vi "LVProjectShortcut_CreateNewWizard_Invoke.vi"(10 "Cluster":T1, 11 "Wizard":T2) -> (3 "Canceled":bool)   [LabVIEW 2017]
uses:
  <resource>/Framework/Providers/API/ItemRef.ctl
  <resource>/Framework/Providers/API/mxLvNIIM.ctl
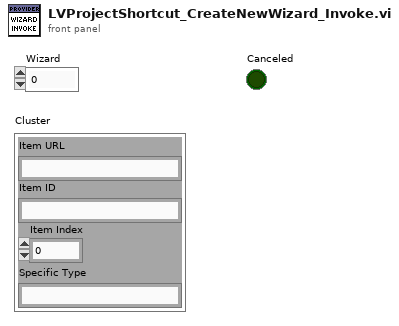
[diagram p1: front panel]
types:
  T1 = typedef "mxLvNIIM.ctl" = cluster{"Item URL":string, "Item ID":string, "Item Index":i32, "Specific Type":string}
  T2 = typedef "ItemRef.ctl" = u64
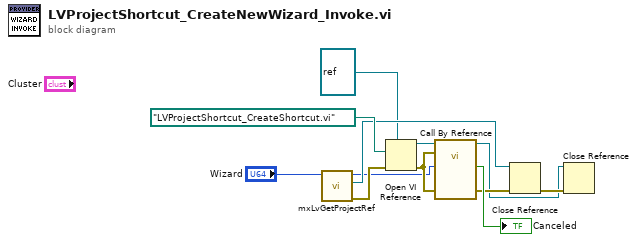
[diagram p0: block diagram]
diagram:
  n1 = call <resource>:"mxLvGetProjectRef.vi"("Item"="Wizard") -> ("error out"=w10:errorcluster, "Project Refnum"=w8:refnum<vi>, "Item"=w1:T2)  [unwired: 8 in]
  n2 = Open VI Reference(type specifier VI Refnum (for type only)=refnum<vi> refnum, vi path=path "LVProjectShortcut_CreateShortcut.vi", error in (no error)=w10) -> (vi reference=w3:refnum<vi>, error out=w9:errorcluster)  [unwired: 3 in]
  n3 = call-by-ref "?"(reference=w3, error in=w9, 6:"error in (no error)"=w9, "Wizard"=w1) -> (reference out=w2:refnum<vi>, "error out"=w5:errorcluster, "Cancelled?"=→"Canceled":bool)  [unwired: 6 in, 1 out]
  n4 = Close Reference(reference=w8, error in (no error)=w5) -> (error out=w7:errorcluster)
  n5 = Close Reference(reference=w2, error in (no error)=w7) -> ()  [unwired: 1 out]
